vi "Lock Front Panel.vi"(8 "error in":errorcluster, 10 "Lock?":bool, 11 "6700 in":refnum<class "6700.lvclass">) -> (0 "error out":errorcluster, 3 "6700 out":refnum<class "6700.lvclass">)   [LabVIEW 2018, in "6700.lvlib" / "6700.lvclass"]
doc: "This VI allows the program to lock out front panel controls or unlock them."
uses:
  6700.lvclass
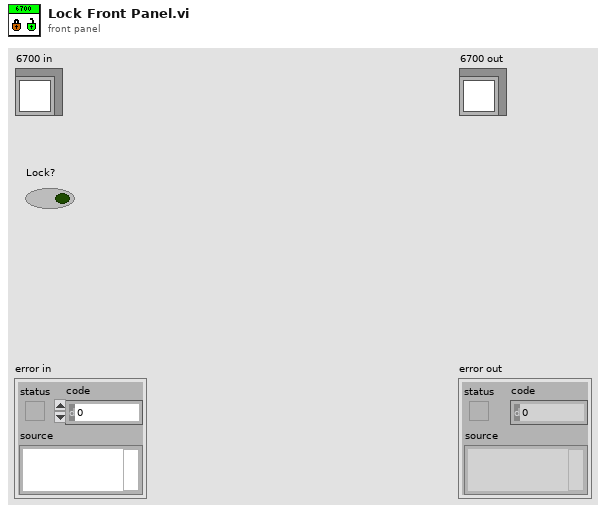
[diagram p1: front panel]
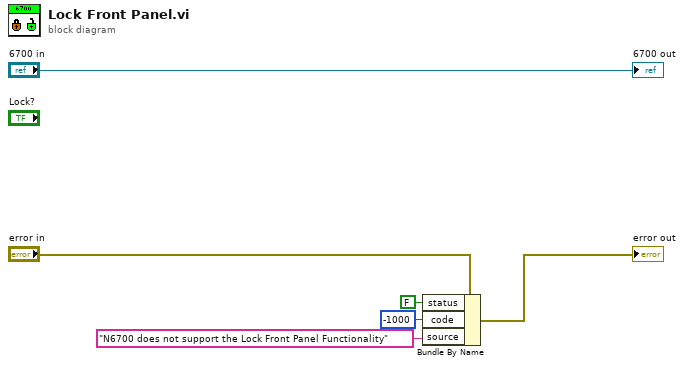
[diagram p0: block diagram]
diagram:
  n1 = Bundle By Name(cluster="error in", "status"=FALSE, "code"=-1000, "source"="N6700 does not support the Lock Front Panel Functionality") -> (→"error out":errorcluster)
  "6700 out" <- "6700 in"
